vi "Change Data Range.vi"(8 "error in":errorcluster, 9 "Minimum":sgl, 10 "Maximum":sgl, 11 "BigMAQ in":refnum<class "BigMAQ.lvclass">) -> (0 "error out":errorcluster, 3 "BigMAQ out":refnum<class "BigMAQ.lvclass">)   [LabVIEW 2019, in "BigMAQ.lvclass"]
uses:
  BigMAQ.lvclass
  BigMAQ.lvclass/BigMAQ.ctl
  <userlib>/_OpenG.lib/md5/md5.llb/MD5 Message Digest (Binary String)__ogtk.vi
  <vilib>/vision/NI_Vision_Development_Module.lvlib
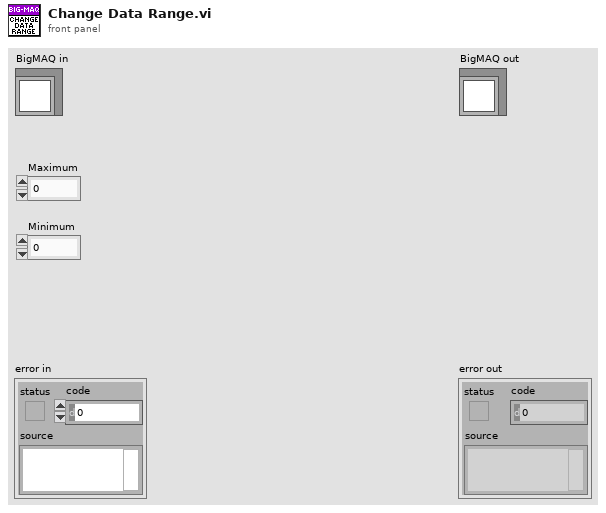
[diagram p1: front panel]
types:
  T1 = typedef "IMAQ Image.ctl" = refnum<image>
  T2 = typedef "Image Type" = u32
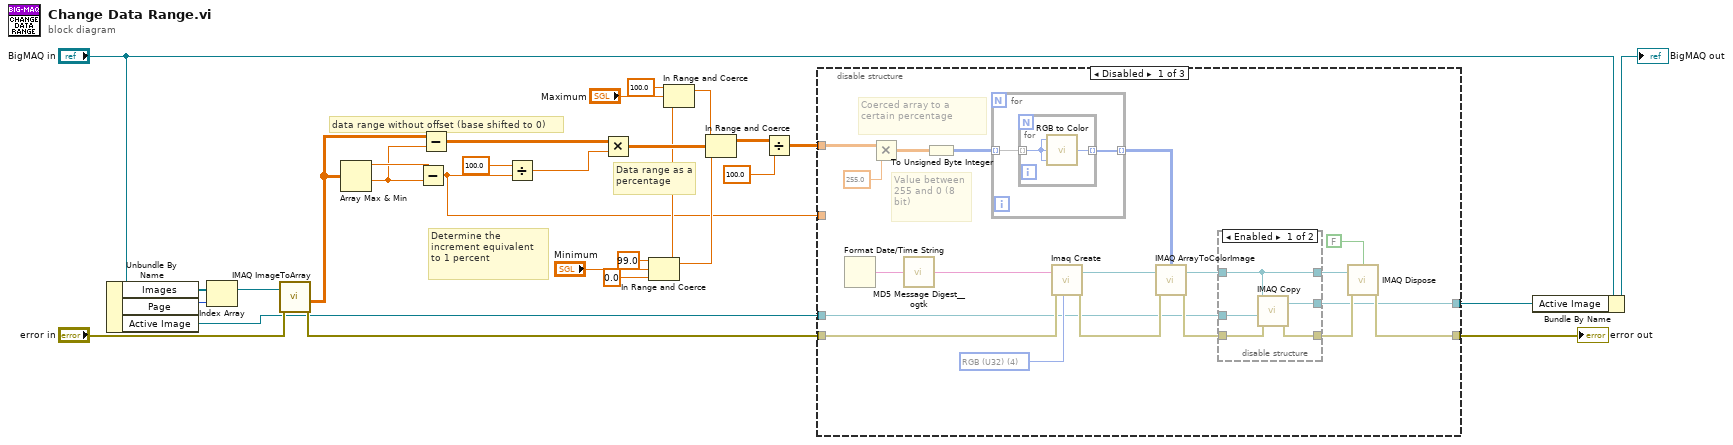
[diagram p0: block diagram]
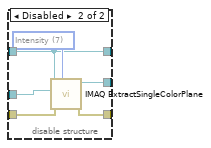
[diagram p2: hidden frame]
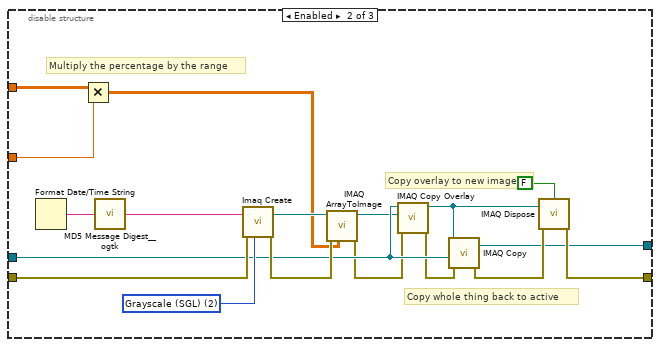
[diagram p3: hidden frame]
diagram:
  # "Determine the increment equivalent to 1 percent"
  # "Data range as a percentage"
  # "data range without offset (base shifted to 0)"
  n1 = Unbundle By Name("BigMAQ in") -> ("Images"=w18:T1[], "Page"=w5:u32, "Active Image"=w1:T1)
  n2 = Index Array(array=w18, index=w5) -> (element=w4:T1)
  n3 = call "IMAQ ImageToArray"("error in (no error)"="error in", "Image"=w4) -> ("Image Pixels (Float)"=w26:sgl[][], "error out"=w15:errorcluster)  [unwired: 2 in, 3 out]
  n4 = Array Max & Min(array=w26) -> (max value=w28:sgl, min value=w25:sgl)  [unwired: 2 out]
  n5 = Subtract(x=w28, y=w25) -> (x-y=w2:sgl)
  n6 = Subtract(x=w26, y=w25) -> (x-y=w23:sgl[][])
  n7 = Divide(x=sgl 100.0, y=w2) -> (x/y=w24:sgl)
  n8 = Multiply(x=w23, y=w24) -> (x*y=w22:sgl[][])
  n9 = In Range and Coerce(upper limit=sgl 99.0, x="Minimum", lower limit=sgl 0.0) -> (coerced(x)=w6:sgl)  [unwired: 1 out]
  n10 = In Range and Coerce(upper limit=sgl 100.0, x="Maximum", lower limit=w6) -> (coerced(x)=w8:sgl)  [unwired: 1 out]
  n11 = In Range and Coerce(upper limit=w8, x=w22, lower limit=w6) -> (coerced(x)=w21:sgl[][])  [unwired: 1 out]
  n12 = Divide(x=w21, y=sgl 100.0 ("Minimum")) -> (x/y=w17:sgl[][])
  n13 = disable-structure shown="Disabled" {
    disable-tunnel: w17 -> [w44 w72 _]
    disable-tunnel: w15 -> [w40 w80 w82]
    disable-tunnel: [w35 w76 w82] -> w14
    disable-tunnel: [w34 w75 w81] -> w13
    disable-tunnel: w1 -> [w29 w67 w81]
    disable-tunnel: w2 -> [_ w71 _]
    frame Disabled {
      w38 = T2 4 items=["Grayscale (U8)", "Grayscale (I16)", "Grayscale (SGL)", "Complex (CSG)", "RGB (U32)", "HSL (U32)", "RGB (U64)", "Grayscale (U16)"] ("Image Type")
      # "Value between 255 and 0 (8 bit)"
      # "Coerced array to a certain percentage"
      n14 = Format Date/Time String() -> (date/time string=w33:string)  [unwired: 3 in]
      n15 = Multiply(x=w44, y=sgl 255.0) -> (x*y=w46:sgl[][])
      n16 = call-poly <userlib>:"MD5 Message Digest__ogtk.vi"("Message"=w33) -> ("MD5 Message Digest"=w32:string)
      n17 = To Unsigned Byte Integer(number=w46) -> (unsigned 8bit integer=w45:u8[][])
      n18 = for {
        tunnel: w45 -> [w60] mode=indexing
        tunnel: [w59] -> w43 mode=indexing
        n19 = for {
          tunnel: w60 -> [w62] mode=indexing
          tunnel: [w61] -> w59 mode=indexing
          n20 = call <vilib>:"RGB to Color.vi"("B"=w62, "G"=w62, "R"=w62) -> ("Color"=w61:u32)
        }
      }
      n21 = call "Imaq Create"("Image Name"=w32, "Image Type"=w38, "error in (no error)"=w40) -> ("New Image"=w41:T1, "error out"=w39:errorcluster)  [unwired: 2 in]
      n22 = call "IMAQ ArrayToColorImage"("Image Pixels (U32)"=w43, "Image"=w41, "error in (no error)"=w39) -> ("Image Out"=w31:T1, "error out"=w42:errorcluster)  [unwired: 2 in]
      n23 = disable-structure shown="Enabled" {
        disable-tunnel: w42 -> [w52 w54]
        disable-tunnel: [w51 w55] -> w36
        disable-tunnel: [w50 w57] -> w34
        disable-tunnel: w29 -> [w49 w58]
        disable-tunnel: w31 -> [w48 w53]
        disable-tunnel: [w48 w53] -> w30
        frame Enabled {
          n24 = call "IMAQ Copy"("error in (no error)"=w52, "Image Dst"=w49, "Image Src"=w48) -> ("error out"=w51:errorcluster, "Image Dst Out"=w50:T1)  [unwired: 3 in]
        }
        frame Disabled {
          w56 = 7 items=["Red", "Green", "Blue", "Hue", "Saturation", "Luminance", "Value", "Intensity"] ("Color Plane")
          n25 = call "IMAQ ExtractSingleColorPlane"("Color Plane"=w56, "error in (no error)"=w54, "Image Dst"=w58, "Image Src"=w53) -> ("error out"=w55:errorcluster, "Image Dst Out"=w57:T1)  [unwired: 6 in]
        }
      }
      n26 = call "IMAQ Dispose"("All Images? (No)"=FALSE, "Image"=w30, "error in (no error)"=w36) -> ("error out"=w35:errorcluster)  [unwired: 3 in]
    }
    frame Enabled {
      w79 = T2 2 items=["Grayscale (U8)", "Grayscale (I16)", "Grayscale (SGL)", "Complex (CSG)", "RGB (U32)", "HSL (U32)", "RGB (U64)", "Grayscale (U16)"] ("Image Type")
      # "Copy whole thing back to active"
      # "Copy overlay to new image"
      # "Multiply the percentage by the range"
      n27 = Format Date/Time String() -> (date/time string=w74:string)  [unwired: 3 in]
      n28 = Multiply(x=w72, y=w71) -> (x*y=w68:sgl[][])
      n29 = call-poly <userlib>:"MD5 Message Digest__ogtk.vi"("Message"=w74) -> ("MD5 Message Digest"=w73:string)
      n30 = call "Imaq Create"("Image Name"=w73, "Image Type"=w79, "error in (no error)"=w80) -> ("New Image"=w69:T1, "error out"=w70:errorcluster)  [unwired: 2 in]
      n31 = call "IMAQ ArrayToImage"("Image Pixels (Float)"=w68, "error in (no error)"=w70, "Image"=w69) -> ("error out"=w64:errorcluster, "Image Out"=w66:T1)  [unwired: 7 in]
      n32 = call "IMAQ Copy Overlay"("error in (no error)"=w64, "Image Dst"=w66, "Image Src"=w67) -> ("error out"=w63:errorcluster, "Image Dst Out"=w65:T1)  [unwired: 7 in]
      n33 = call "IMAQ Copy"("error in (no error)"=w63, "Image Dst"=w67, "Image Src"=w65) -> ("error out"=w77:errorcluster, "Image Dst Out"=w75:T1)  [unwired: 3 in]
      n34 = call "IMAQ Dispose"("All Images? (No)"=FALSE, "Image"=w65, "error in (no error)"=w77) -> ("error out"=w76:errorcluster)  [unwired: 3 in]
    }
    frame Disabled {
    }
  }
  "error out" <- w14
  n35 = Bundle By Name(cluster="BigMAQ in", "Active Image"=w13) -> (→"BigMAQ out":refnum<class "BigMAQ.lvclass">)
